vi "set_I_channel.vi"(8 "error in (no error)":errorcluster, 9 "current":dbl min=0.0 max=5.0, 10 "channel":T1=enum."1", 11 "Motech-pps-1200 in":refnum<class "Motech-pps-1200.lvclass">) -> (0 "error out":errorcluster, 3 "Motech-pps-1200 out":refnum<class "Motech-pps-1200.lvclass">)   [LabVIEW 2017, in "Motech-pps-1200.lvclass"]
uses:
  Motech-pps-1200.lvclass
  subVI/motech_power_supply/types/channels_enum.ctl
  Motech-pps-1200.lvclass/Motech-pps-1200.ctl
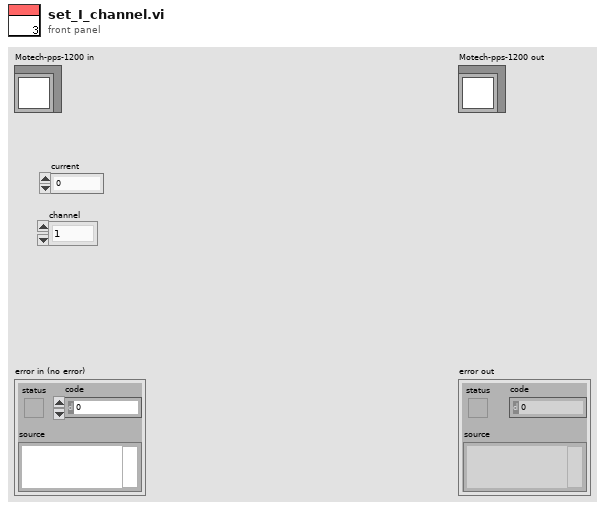
[diagram p1: front panel]
types:
  T1 = typedef "channels_enum.ctl" = enum16{"0", "1", "2"}
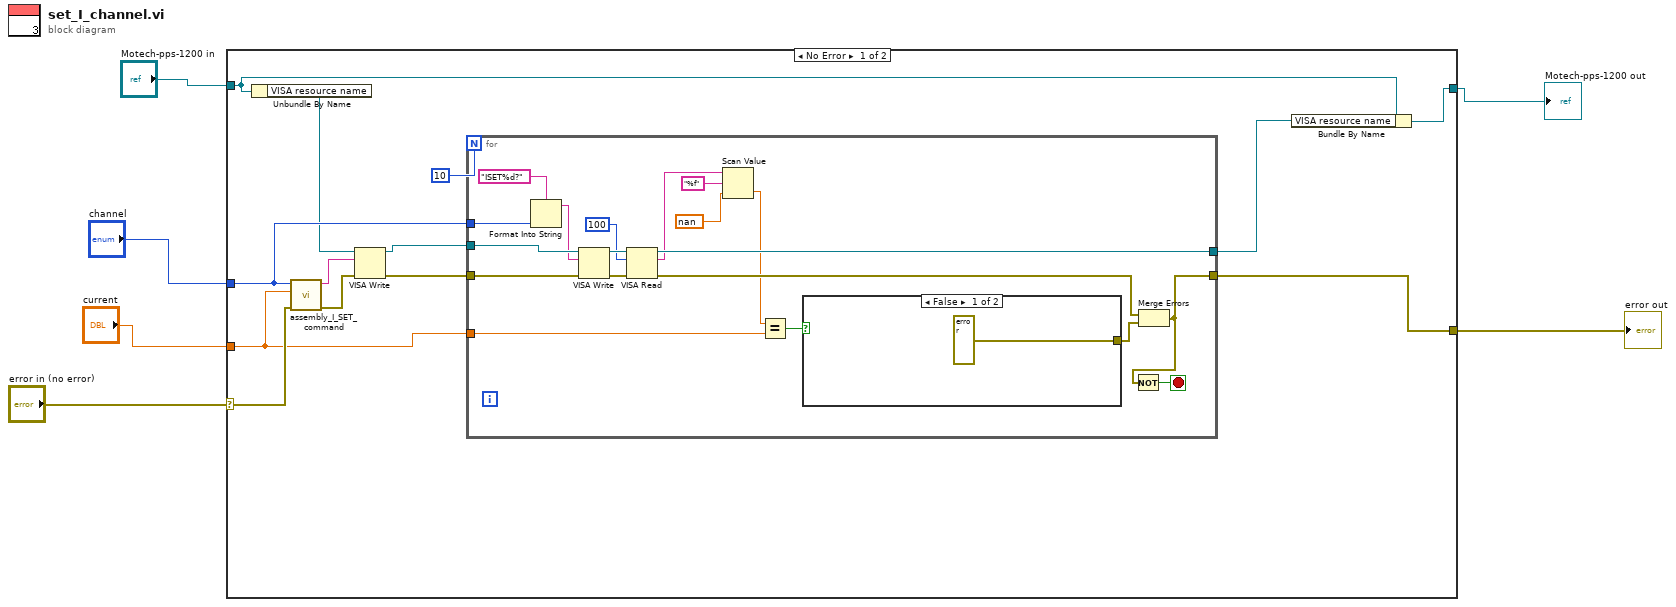
[diagram p0: block diagram]
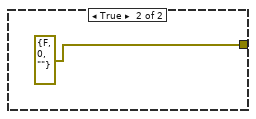
[diagram p2: hidden frame]
diagram:
  n1 = case shown="No Error" "error in (no error)" {
    selector: "error in (no error)" -> [w13 w42]
    tunnel: [w16 w42] -> w5
    tunnel: "channel" -> [w15 _]
    tunnel: "current" -> [w12 _]
    tunnel: [w9 w41] -> w3
    tunnel: "Motech-pps-1200 in" -> [w11 w41]
    frame No Error {
      n2 = Unbundle By Name(w11) -> ("VISA resource name"=w7:refnum<visa-resource-name>)
      n3 = call "assembly_I_SET_command.vi"("error_in"=w13, "curr"=w12, "channel"=w15) -> ("error_out"=w14:errorcluster, "command"=w19:string)  [unwired: 7 in]
      n4 = VISA Write(VISA resource name=w7, write buffer=w19, error in (no error)=w14) -> (VISA resource name out=w18:refnum<visa-resource-name>, error out=w17:errorcluster)  [unwired: 1 out]
      n5 = for {
        N: 10 -> [_]
        tunnel: w18 -> [w38]
        tunnel: w17 -> [w37]
        tunnel: [w33] -> w10
        tunnel: [w25] -> w16
        tunnel: w12 -> [w29]
        tunnel: w15 -> [w22]
        stop <- w26 stop-if-true
        n6 = Format Into String(format string="ISET%d?" ("write buffer"), w22) -> (resulting string=w21:string)  [unwired: 2 in, 1 out]
        n7 = VISA Write(VISA resource name=w38, write buffer=w21, error in (no error)=w37) -> (VISA resource name out=w36:refnum<visa-resource-name>, error out=w35:errorcluster)  [unwired: 1 out]
        n8 = VISA Read(VISA resource name=w36, byte count=u32 100, error in (no error)=w35) -> (VISA resource name out=w33:refnum<visa-resource-name>, read buffer=w31:string, error out=w27:errorcluster)  [unwired: 1 out]
        n9 = Scan Value(string=w31, format string="%f", default (0 dbl)=nan) -> (value=w20:dbl)  [unwired: 1 out]
        n10 = Equal?(x=w20, y=w29) -> (x = y?=w30:bool)
        n11 = case shown="False" w30 {
          tunnel: [errorcluster {"status"=TRUE, "code"=1, "source"="Не удалось установить требуемое значение тока"} ("error constant") errorcluster {"status"=FALSE, "code"=0, "source"=""} ("error constant")] -> w28
          frame False {
          }
          frame True {
          }
        }
        n12 = Merge Errors(w27, w28) -> (w25:errorcluster)
        n13 = Not(x=w25) -> (.not. x?=w26:bool)
      }
      n14 = Bundle By Name(cluster=w11, "VISA resource name"=w10) -> (w9:refnum<class "Motech-pps-1200.lvclass">)
    }
    frame Error {
    }
  }
  "error out" <- w5
  "Motech-pps-1200 out" <- w3
